vi "readIMUData.vi"(2 "IMU Config In":T1={"Accelerometer Bias"=[0, 0, 0], "Accelerometer Scale"=0, "Gyro Bias"=[0, 0, 0], "Gyro Scale"=0}, 3 "SPI Config In":T2) -> (0 "Data Out":T3, 1 "SPI Config Out":T2)   [LabVIEW 2019]
uses:
  SPI/SPI Config.ctl
  IMU Config.ctl
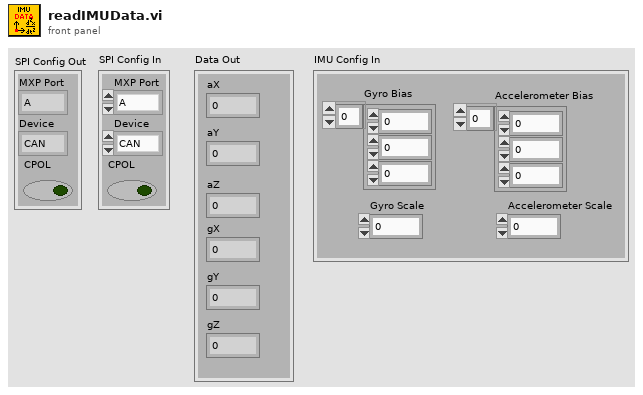
[diagram p1: front panel]
types:
  T1 = typedef "IMU Config.ctl" = cluster{"Accelerometer Bias":i16[], "Accelerometer Scale":i16, "Gyro Bias":i16[], "Gyro Scale":i16}
  T2 = typedef "SPI Config.ctl" = cluster{"MXP Port":enum16{"A", "B"}, "Device":enum16{"CAN", "ENC", "IMU1", "IMU2"}, "CPOL":bool}
  T3 = cluster{fxp<+/-,32,16>, fxp<+/-,32,16>, fxp<+/-,32,16>, fxp<+/-,32,16>, fxp<+/-,32,16>, fxp<+/-,32,16>}
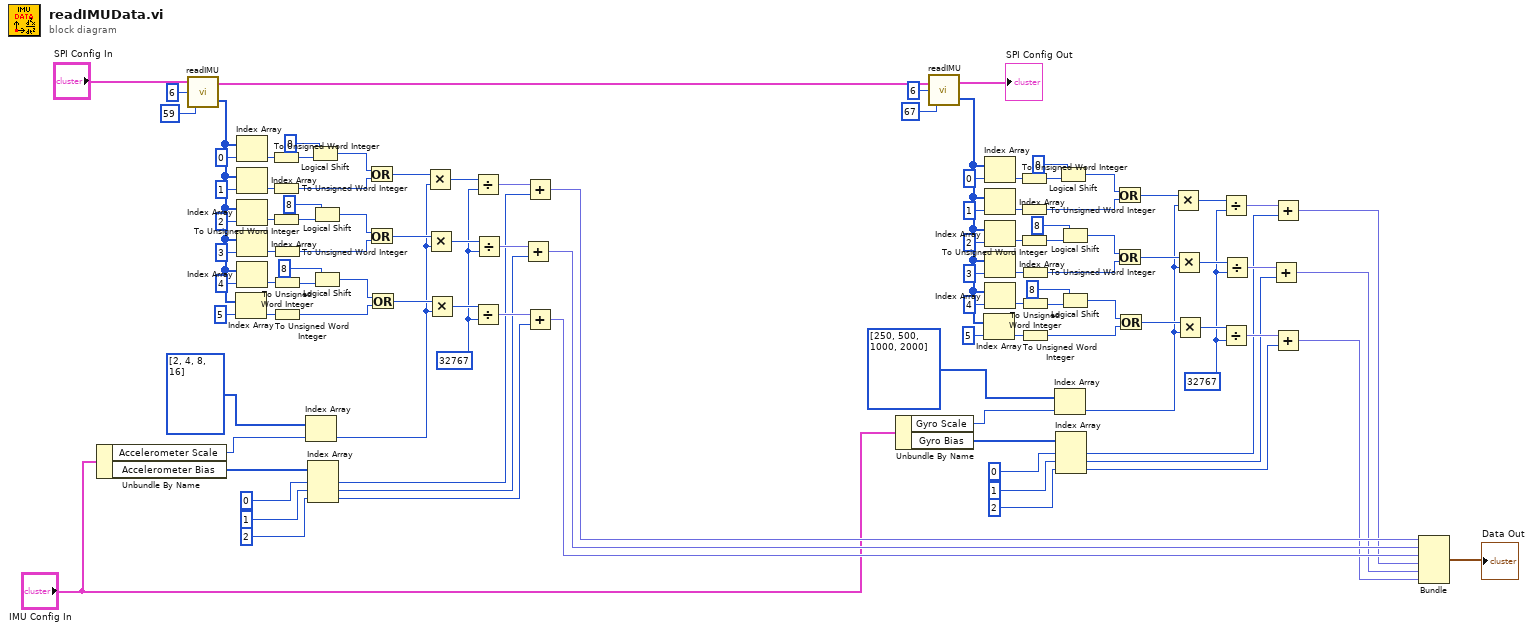
[diagram p0: block diagram]
diagram:
  w22 = i16 32767 ("y")
  w65 = i16 32767 ("y")
  n1 = Unbundle By Name("IMU Config In") -> ("Accelerometer Scale"=w6:i16, "Accelerometer Bias"=w9:i16[])
  n2 = call "readIMU.vi"("Address"=u8 59, "Frames to Read"=u8 6, "SPI Config In"="SPI Config In") -> ("Data Read"=w99:u8[], "SPI Config Out"=w102:T2)
  n3 = Index Array(array=w99, index=5) -> (element=w87:u8)
  n4 = Index Array(array=w99, index=0) -> (element=w92:u8)
  n5 = Index Array(array=w99, index=1) -> (element=w91:u8)
  n6 = Index Array(array=w99, index=2) -> (element=w90:u8)
  n7 = Index Array(array=w99, index=3) -> (element=w89:u8)
  n8 = Index Array(array=w99, index=4) -> (element=w88:u8)
  n9 = To Unsigned Word Integer(number=w92) -> (unsigned 16bit integer=w86:u16)
  n10 = To Unsigned Word Integer(number=w91) -> (unsigned 16bit integer=w79:u16)
  n11 = To Unsigned Word Integer(number=w90) -> (unsigned 16bit integer=w84:u16)
  n12 = To Unsigned Word Integer(number=w89) -> (unsigned 16bit integer=w77:u16)
  n13 = To Unsigned Word Integer(number=w88) -> (unsigned 16bit integer=w82:u16)
  n14 = To Unsigned Word Integer(number=w87) -> (unsigned 16bit integer=w75:u16)
  n15 = Index Array(array=u16[] [2, 4, 8, 16], index=w6) -> (element=w4:u16)
  n16 = Index Array(array=w9, index #1=0 ("index"), index #2=1 ("index"), index #3=2 ("index")) -> (element #1=w61:i16, element #2=w60:i16, element #3=w59:i16)
  n17 = Logical Shift(y=i16 8, x=w86) -> (x << y=w80:u16)
  n18 = Logical Shift(y=i16 8, x=w84) -> (x << y=w78:u16)
  n19 = Logical Shift(y=i16 8, x=w82) -> (x << y=w76:u16)
  n20 = Or(x=w80, y=w79) -> (x .or. y?=w74:u16)
  n21 = Or(x=w78, y=w77) -> (x .or. y?=w73:u16)
  n22 = Or(x=w76, y=w75) -> (x .or. y?=w72:u16)
  n23 = Multiply(x=w74, y=w4) -> (x*y=w68:u16)
  n24 = Multiply(x=w73, y=w4) -> (x*y=w67:u16)
  n25 = Multiply(x=w72, y=w4) -> (x*y=w66:u16)
  n26 = Divide(x=w68, y=w65) -> (x/y=w64:fxp<+/-,32,16>)
  n27 = Divide(x=w66, y=w65) -> (x/y=w62:fxp<+/-,32,16>)
  n28 = Divide(x=w67, y=w65) -> (x/y=w63:fxp<+/-,32,16>)
  n29 = Add(x=w63, y=w60) -> (x+y=w57:fxp<+/-,32,16>)
  n30 = Add(x=w64, y=w61) -> (x+y=w58:fxp<+/-,32,16>)
  n31 = Add(x=w62, y=w59) -> (x+y=w56:fxp<+/-,32,16>)
  n32 = Unbundle By Name("IMU Config In") -> ("Gyro Scale"=w3:i16, "Gyro Bias"=w8:i16[])
  n33 = call "readIMU.vi"("Address"=u8 67, "Frames to Read"=u8 6, "SPI Config In"=w102) -> ("Data Read"=w15:u8[], "SPI Config Out"=→"SPI Config Out":T2)
  n34 = Index Array(array=w15, index=5) -> (element=w44:u8)
  n35 = Index Array(array=w15, index=0) -> (element=w49:u8)
  n36 = Index Array(array=w15, index=1) -> (element=w48:u8)
  n37 = Index Array(array=w15, index=2) -> (element=w47:u8)
  n38 = Index Array(array=w15, index=3) -> (element=w46:u8)
  n39 = Index Array(array=w15, index=4) -> (element=w45:u8)
  n40 = To Unsigned Word Integer(number=w49) -> (unsigned 16bit integer=w43:u16)
  n41 = To Unsigned Word Integer(number=w48) -> (unsigned 16bit integer=w36:u16)
  n42 = To Unsigned Word Integer(number=w47) -> (unsigned 16bit integer=w41:u16)
  n43 = To Unsigned Word Integer(number=w46) -> (unsigned 16bit integer=w34:u16)
  n44 = To Unsigned Word Integer(number=w45) -> (unsigned 16bit integer=w39:u16)
  n45 = To Unsigned Word Integer(number=w44) -> (unsigned 16bit integer=w32:u16)
  n46 = Index Array(array=u16[] [250, 500, 1000, 2000], index=w3) -> (element=w1:u16)
  n47 = Index Array(array=w8, index #1=0 ("index"), index #2=1 ("index"), index #3=2 ("index")) -> (element #1=w18:i16, element #2=w17:i16, element #3=w16:i16)
  n48 = Logical Shift(y=i16 8, x=w43) -> (x << y=w37:u16)
  n49 = Logical Shift(y=i16 8, x=w41) -> (x << y=w35:u16)
  n50 = Logical Shift(y=i16 8, x=w39) -> (x << y=w33:u16)
  n51 = Or(x=w37, y=w36) -> (x .or. y?=w31:u16)
  n52 = Or(x=w35, y=w34) -> (x .or. y?=w30:u16)
  n53 = Or(x=w33, y=w32) -> (x .or. y?=w29:u16)
  n54 = Multiply(x=w31, y=w1) -> (x*y=w25:u16)
  n55 = Multiply(x=w30, y=w1) -> (x*y=w24:u16)
  n56 = Multiply(x=w29, y=w1) -> (x*y=w23:u16)
  n57 = Divide(x=w25, y=w22) -> (x/y=w21:fxp<+/-,32,16>)
  n58 = Divide(x=w23, y=w22) -> (x/y=w19:fxp<+/-,32,16>)
  n59 = Divide(x=w24, y=w22) -> (x/y=w20:fxp<+/-,32,16>)
  n60 = Add(x=w20, y=w17) -> (x+y=w12:fxp<+/-,32,16>)
  n61 = Add(x=w21, y=w18) -> (x+y=w13:fxp<+/-,32,16>)
  n62 = Add(x=w19, y=w16) -> (x+y=w11:fxp<+/-,32,16>)
  n63 = Bundle(w58, w57, w56, w13, w12, w11) -> (→"Data Out":T3)  [unwired: 1 in]
